vi "Galvo Signals counts.vi"(10 "Galvo signal readed in":u32, 11 "output valid? in":bool) -> (3 "Galvo signal readed out":u32)   [LabVIEW 2015]
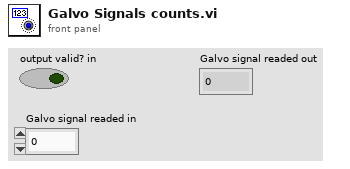
[diagram p1: front panel]
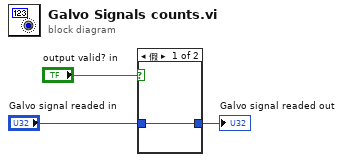
[diagram p0: block diagram]
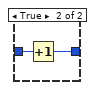
[diagram p2: hidden frame]
diagram:
  n1 = case shown="假" "output valid? in" {
    tunnel: "Galvo signal readed in" -> [w4 w6]
    tunnel: [w4 w5] -> w3
    frame False {
    }
    frame True {
      n2 = Increment(x=w6) -> (x+1=w5:u32)
    }
  }
  "Galvo signal readed out" <- w3
